vi "Toroidal_power_supply_check.vi"(3 "error in":errorcluster, 4 "Step Number in":i32, 5 "Data in":T1) -> (0 "error out":errorcluster, 1 "Step Number out":i32, 2 "Data out":T1)   [LabVIEW 2017, in "Steps.lvlib"]
uses:
  Steps.lvlib
  Type_Defs/Data.ctl
  Type_Defs/Diagnostics.ctl
  Type_Defs/Systems.ctl
panel:
  out "Power Supply 2":bool=TRUE
  in  "Step Back":bool
  in  "Continue":bool
  out "Power Supply 1":bool=TRUE
  # "Options"
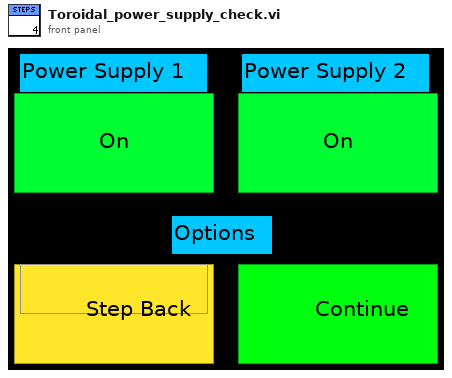
[diagram p1: front panel]
types:
  T1 = typedef "Data.ctl" = cluster{"User Name":string, "Experiment Number":i32, "Start Time":timestamp, "Data":dbl[], "Step Number":i32, "Step Instructions":string, "Diagnostics":T2, "Experiment Purpose":string, "Experiment State":enum16{"Off", "Setting Up", "Ready", "In Progress", "Shutting Down"}, "Systems":T3, "Vacuum Pressure":dbl, "Fieldpoints":cluster{"System Boolean Fieldpoints":cluster{"Compressed Air":refnum<k21>, "T-20kV Power Switch":refnum<k21>, "T-Rectifier":refnum<k21>, "Engage Interlock":refnum<k21>, "Ventilator":refnum<k21>, "Magnetron":refnum<k21>, "H-20kV Power Switch":refnum<k21>, "H-Rectifier":refnum<k21>, "Main Water Pump":refnum<k21>, "WEGA Water Pump":refnum<k21>, "Gas Inlet Valves":refnum<k21>}, "Step Fieldpoints":cluster{"Exhaust Ventillator":refnum<k21>, "Compressed Air":refnum<k21>, "Water Pressure":refnum<k21>, "Interlock":refnum<k21>, "Toroidal Power Supply 1":refnum<k21>, "Toroidal Power Supply 2":refnum<k21>, "Toroidal Rectifier":refnum<k21>, "Helical Power Supply":refnum<k21>, "Helical Rectifier":refnum<k21>, "6kW Magnetron Standby":refnum<k21>, "20kW Magnetron Standby":refnum<k21>}}, "Pressure History":cluster{"Seconds into Experiment":i32[], "Pressure Data":dbl[]}, "Time Computer Control":dbl[], "Toroidal Voltage Computer Control":dbl[], "Helical Voltage Computer Control":dbl[], "Toroidal Current":dbl[], "Toroidal Voltage":dbl[], "Toroidal Current Set Point":dbl[], "Helical Current Set Point":dbl[], "Helical Voltage":dbl[], "Helical Current":dbl[]}
  T2 = typedef "Diagnostics.ctl" = cluster{"Langmuir Probe":bool, "Rogowski 1":bool, "Rogowski 2":bool, "Rogowski 3":bool, "B-dot 1":bool, "B-dot 2":bool}
  T3 = typedef "Systems.ctl" = cluster{"Compressed Air":bool, "T-20kV Power Switch":bool, "T-Rectifier":bool, "Engage Interlock":bool, "Ventilator":bool, "Magnetron":bool, "H-20kV Power Switch":bool, "H-Rectifier":bool, "Main Water Pump":bool, "WEGA Water Pump":bool, "Gas Inlet Valves":bool}
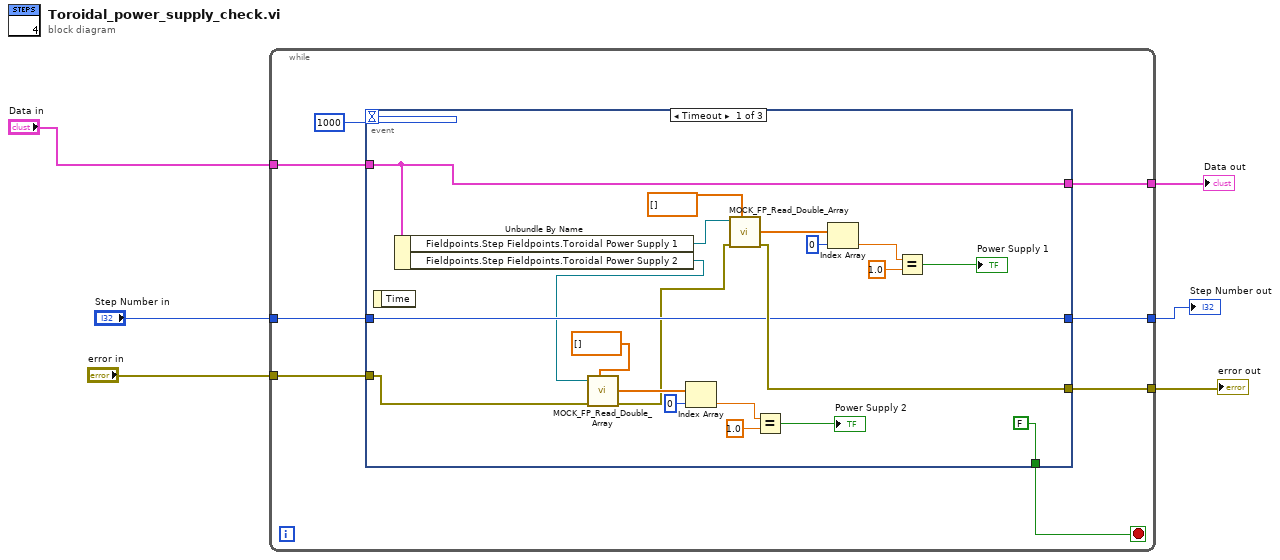
[diagram p0: block diagram]
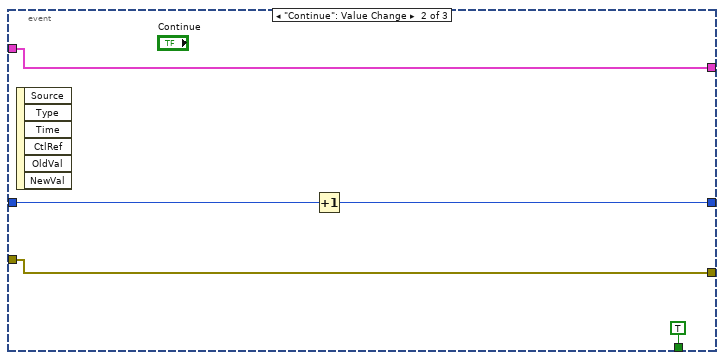
[diagram p2: hidden frame]
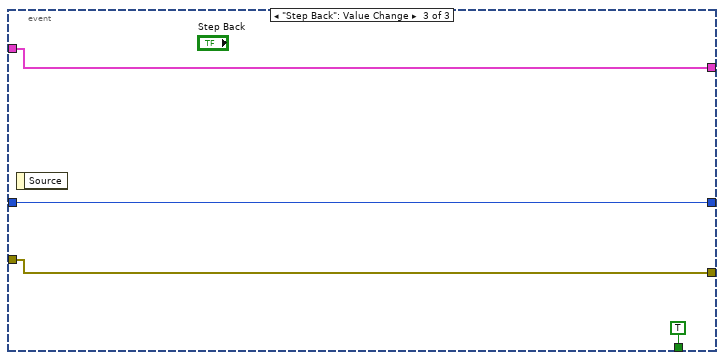
[diagram p3: hidden frame]
diagram:
  n1 = while {
    tunnel: "error in" -> [w13]
    tunnel: [w12] -> w5
    tunnel: [w10] -> w4
    tunnel: "Data in" -> [w9]
    tunnel: [w8] -> w2
    tunnel: "Step Number in" -> [w7]
    stop <- w11 stop-if-true
    n2 = event shown="[0] Timeout" {
      selector: _ -> [_ _ _]
      dyn-events: _ -> [_ _ _]
      timeout: 1000 -> [_ _ _]
      tunnel: w13 -> [w17 w38 w42]
      tunnel: [w30 w38 w42] -> w12
      tunnel: [FALSE TRUE TRUE] -> w11
      tunnel: [w28 w39 w43] -> w10
      tunnel: w9 -> [w28 w39 w43]
      tunnel: [w27 w36 w41] -> w8
      tunnel: w7 -> [w27 w37 w41]
      event Timeout {
        n3 = event-data() -> ()  [unwired: 1 in, 1 out]
        n4 = Unbundle By Name(w28) -> ("Fieldpoints.Step Fieldpoints.Toroidal Power Supply 1"=w24:refnum<k21>, "Fieldpoints.Step Fieldpoints.Toroidal Power Supply 2"=w15:refnum<k21>)
        n5 = call "MOCK_FP_Read_Double_Array.vi"("Type"=dbl[] [], "error in"=w17, "FieldPoint IO Point In"=w15) -> ("error out"=w16:errorcluster, "Array"=w23:dbl[])  [unwired: 5 in, 2 out]
        n6 = Index Array(array=w23, index=0) -> (element=w21:dbl)
        n7 = call "MOCK_FP_Read_Double_Array.vi"("Type"=dbl[] [], "error in"=w16, "FieldPoint IO Point In"=w24) -> ("error out"=w30:errorcluster, "Array"=w34:dbl[])  [unwired: 5 in, 2 out]
        n8 = Equal?(x=w21, y=1.0) -> (x = y?=→"Power Supply 2":bool)
        n9 = Index Array(array=w34, index=0) -> (element=w32:dbl)
        n10 = Equal?(x=w32, y=1.0) -> (x = y?=→"Power Supply 1":bool)
      }
      event "Continue": Value Change {
        n11 = event-data() -> ()  [unwired: 1 in, 6 out]
        n12 = Increment(x=w37) -> (x+1=w36:i32)
      }
      event "Step Back": Value Change {
        n13 = event-data() -> ()  [unwired: 1 in, 1 out]
      }
    }
  }
  "error out" <- w5
  "Data out" <- w4
  "Step Number out" <- w2
